vi "Create Data Channels.vi"(8 "error in":errorcluster, 11 "Node in":refnum<class "BLS Chiller Template.lvclass">) -> (0 "error out":errorcluster, 3 "Node out":refnum<class "BLS Chiller Template.lvclass">)   [LabVIEW 2023, in "BLS Chiller Template.lvlib" / "BLS Chiller Template.lvclass"]
uses:
  BLS Chiller Template.lvclass
  BLS Chiller Template.lvclass/BLS Chiller Template.ctl
  <vilib>/ADAS Replay HIL/Template Node/Plugin/Template Node/Template Node.lvclass
  bls-capabilities/src/Capabilities/High Level Capabilities/Chiller/Chiller.lvclass
  C:/Program Files/National Instruments/LabVIEW 2023/vi.lib/ADAS Replay HIL/Template Node/Plugin/Template Node/Template Node.lvclass
  C:/Program Files/National Instruments/ADAS Replay HIL/EVO SDK/Linux RT/evoLabVIEWAPI/evoBlockPlugin.lvlibp/evoBlockPlugin/BlockPluginInterface.2020.1/BlockPluginInterface.2020.1.lvclass
  C:/Users/amomin/BLS/bls-chiller-plugin-template/Plugin/BLS Chiller Template/BLS Chiller Template.lvclass
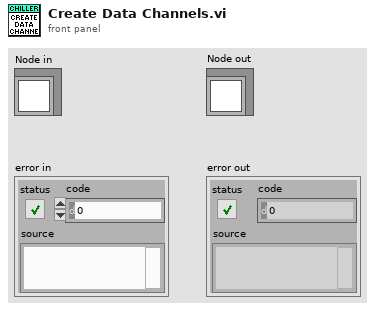
[diagram p1: front panel]
types:
  T1 = typedef "BLS Chiller Template.lvlib/BLS Chiller Template.lvclass/Configuration Params.ctl" = cluster{"Common":T2, "Amount of Channels":u32, "Address":string}
  T2 = typedef "Template Node.lvlib/Template Node.lvclass/Common Configuration Params.ctl" = cluster{"Iteration Interval (s)":dbl, "T0 (ns)":u64, "Priority":i32, "Processor":i32, "Wait in Ready State":bool}
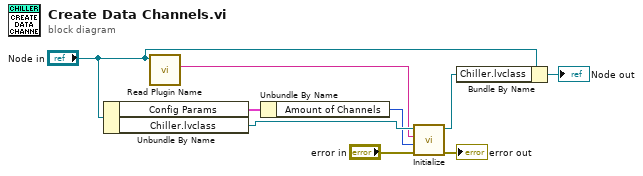
[diagram p0: block diagram]
diagram:
  n1 = Unbundle By Name("Node in") -> ("Config Params"=w9:T1, "Chiller.lvclass"=w5:refnum<class "Chiller.lvclass">)
  n2 = call <vilib>:"Read Plugin Name.vi"("Template Node in"="Node in") -> ("Plugin Name"=w1:string)  [unwired: 8 in, 2 out]
  n3 = Unbundle By Name(w9) -> ("Amount of Channels"=w2:u32)
  n4 = call-dynamic "Initialize.vi"("error in"="error in", "Number of Channels"=w2, "Instance Name"=w1, "Chiller in"=w5) -> ("error out"=→"error out":errorcluster, "Chiller out"=w6:refnum<class "Chiller.lvclass">)  [unwired: 6 in]
  n5 = Bundle By Name(cluster="Node in", "Chiller.lvclass"=w6) -> (→"Node out":refnum<class "BLS Chiller Template.lvclass">)
